vi "ChangeLight.vi"(0 "object in":refnum<class "TrafficLight.lvclass">, 5 "Error In":errorcluster) -> (14 "object out":refnum<class "TrafficLight.lvclass">, 19 "Error Out":errorcluster)   [LabVIEW 2024, in "TrafficLight.lvclass"]
doc: "Trigger a state change. This method only triggers the current state to change state. Therefore this method does not implement any logic to change states."
uses:
  TrafficLight.lvclass
  TrafficLight.lvclass/TrafficLight.ctl
  State_interface/State.lvclass
panel:
  # "Connector Pane"
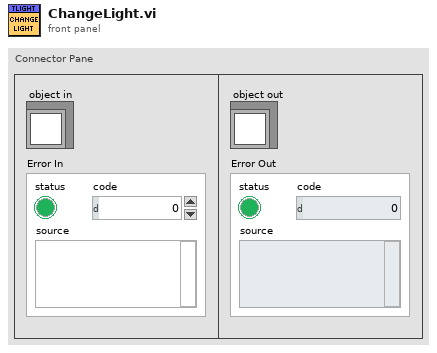
[diagram p1: front panel]
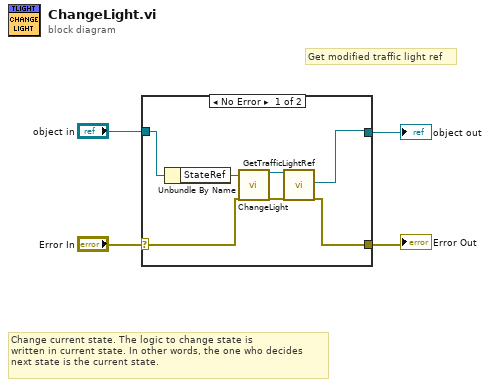
[diagram p0: block diagram]
diagram:
  # "Get modified traffic light ref"
  # "Change current state. The logic to change state is\nwritten in current state. In other words, the one who decides\nnext state is the current state."
  n1 = case shown="No Error" "Error In" {
    selector: "Error In" -> [w9 w13]
    tunnel: [w6 w13] -> w3
    tunnel: [w7 w12] -> w1
    tunnel: "object in" -> [w11 w12]
    frame No Error {
      n2 = Unbundle By Name(w11) -> ("StateRef"=w10:refnum<class "State.lvclass">)
      n3 = call-dynamic "ChangeLight.vi"("object in"=w10, "Error In"=w9) -> ("object out"=w5:refnum<class "State.lvclass">, "Error Out"=w8:errorcluster)  [unwired: 16 in]
      n4 = call-dynamic "GetTrafficLightRef.vi"("object in"=w5, "Error In"=w8) -> ("TrafficLightRef"=w7:refnum<class "TrafficLight.lvclass">, "Error Out"=w6:errorcluster)  [unwired: 15 in, 1 out]
    }
    frame Error {
    }
  }
  "Error Out" <- w3
  "object out" <- w1
